vi "InOutdegree.vi"(9 "DAG in":refnum<class "DAG.lvclass">) -> (4 "outdegree":i32[](array[numeric]), 5 "indegree":i32[](array[numeric]))   [LabVIEW 2014, in "DAG.lvclass"]
uses:
  DAG.lvclass
  DAG.lvclass/DAG.ctl
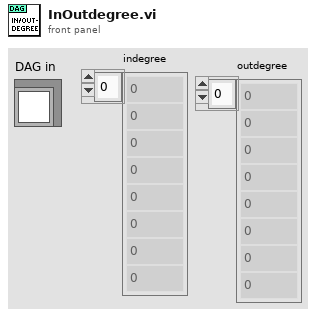
[diagram p1: front panel]
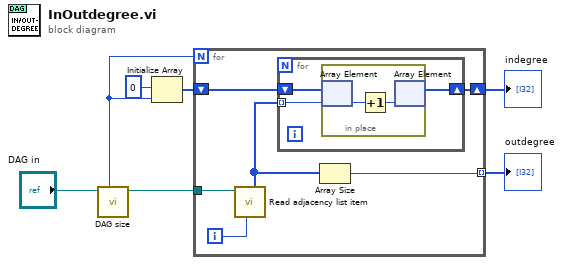
[diagram p0: block diagram]
diagram:
  n1 = call "DAG size.vi"("DAG in"="DAG in") -> ("DAG out"=w3:refnum<class "DAG.lvclass">, "vertices"=w6:i32)  [unwired: 6 in, 1 out]
  n2 = Initialize Array(0, w6) -> (w4:i32[])
  n3 = for {
    N: w6 -> [_]
    shift-right: [w10] -> w2
    shift-left: w4 -> [w11]
    tunnel: w3 -> [w13]
    tunnel: [w9] -> w1 mode=indexing
    i -> [w12]
    n4 = call "Read adjacency list item.vi"("vertex"=w12, "DAG in"=w13) -> ("edge list"=w8:i32[])  [unwired: 6 in, 1 out]
    n5 = for {
      shift-right: [w14] -> w10
      shift-left: w11 -> [w16]
      tunnel: w8 -> [w15] mode=indexing
      n6 = in-place {
        n7 = in-place-array #1(w16, w15) -> (w18:i32)
        n8 = Increment(x=w18) -> (x+1=w17:i32)
        n9 = in-place-array #1(w17) -> (w14:i32[])  [unwired: 1 out]
      }
    }
    n10 = Array Size(array=w8) -> (size(s)=w9:i32)
  }
  "indegree" <- w2
  "outdegree" <- w1
